vi "General setup bundler-Boolean.vi"(8 "error in (no error)":errorcluster, 9 "Boolean":T2, 10 "Section":string, 11 "Setup.ini ref":T1) -> (0 "error out":errorcluster, 3 "Setup.ini ref":T1)   [LabVIEW 2020]
uses:
  Typedefs/Ini file interface (Boolean).ctl
  <vilib>/Utility/config.llb/Config Data RefNum.ctl
  Typedefs/fgv_actions.ctl
  Global Variables/General Globals.vi
  <vilib>/Utility/config.llb/NI_LVConfig.lvlib
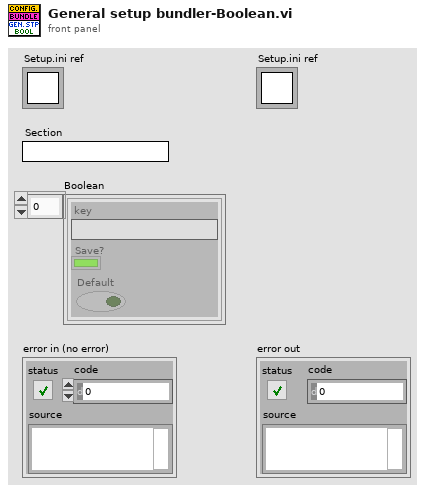
[diagram p1: front panel]
types:
  T1 = typedef "NI_LVConfig.lvlib/Config Data RefNum.ctl" = refnum<k1>
  T2 = typedef "Ini file interface (Boolean).ctl" = cluster{"key":string, "Save?":bool, "Default":bool}[]
  T3 = typedef "fgv_actions.ctl" = enum16{"Get", "Set"}
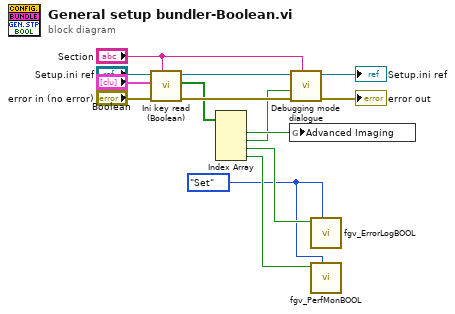
[diagram p0: block diagram]
diagram:
  w1 = fgv_actions."Set" ("FGV Actions")
  n1 = call "Ini key read (Boolean).vi"("Section"="Section", "error in (no error)"="error in (no error)", "Parameter names & setup"="Boolean", "Ini file refnum in"="Setup.ini ref") -> ("error out"=→"error out":errorcluster, "Value read/used"=w10:bool[], "Ini file refnum out"=w8:T1)  [unwired: 5 in]
  n2 = Index Array(array=w10) -> (element #1=w5:bool, element #2=w4:bool, element #3=w3:bool, element #4=w2:bool)  [unwired: 4 in]
  n3 = global write "General Globals.vi" "Advanced Imaging"(w5) -> ()
  n4 = call "Debugging mode dialogue.vi"("Section"="Section", "Loaded value for \"DevPC - No hardware\""=w4, "Setup.ini ref"=w8) -> ("Setup.ini ref"=→"Setup.ini ref":T1)  [unwired: 8 in]
  n5 = call "fgv_ErrorLogBOOL.vi"("FGV Actions"=w1, "Error Logging ON [IN] ?"=w3) -> ()  [unwired: 8 in, 2 out]
  n6 = call "fgv_PerfMonBOOL.vi"("FGV Actions"=w1, "Perf Mon [IN]"=w2) -> ()  [unwired: 8 in, 2 out]
